vi "clFile_writeToFile.vi"(8 "filename (use dialog)":path, 11 "clFile.lvclass":refnum<class "clFile.lvclass">) -> (3 "no Error":bool)   [LabVIEW 2016, in "vi_lib.lvlib" / "clFile.lvclass"]
uses:
  clFile.lvclass
  clFile.lvclass/clFile.ctl
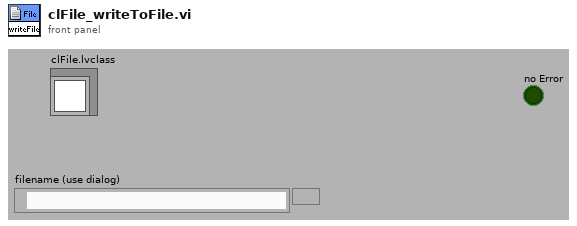
[diagram p1: front panel]
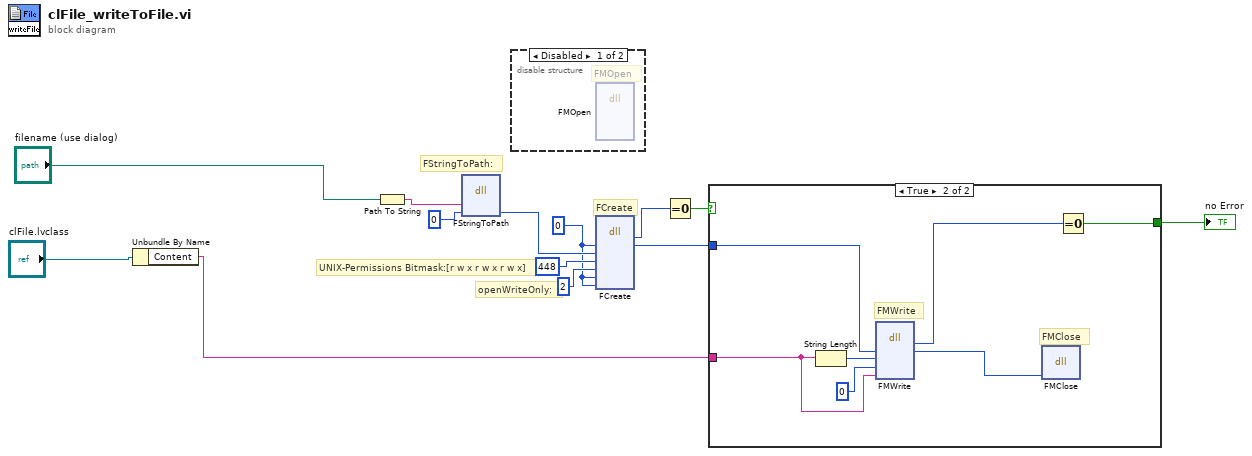
[diagram p0: block diagram]
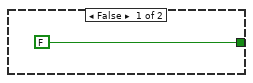
[diagram p2: hidden frame]
diagram:
  w4 = 0 ("denyMode")
  # "FCreate"
  # "FStringToPath:"
  # "UNIX-Permissions Bitmask:[r w x r w x r w x]"
  # "openWriteOnly:"
  n1 = Unbundle By Name("clFile.lvclass") -> ("Content"=w12:string)
  n2 = Path To String(path="filename (use dialog)") -> (string=w8:string)
  n3 = dll-call lib="LabVIEW" fn="FStringToPath"("path"=w8, "pid"=u32 0) -> ("pid"=w7:u32)  [unwired: 4 in, 3 out]
  n4 = disable-structure shown="Disabled" {
    frame Disabled {
      # "FMOpen"
      n5 = dll-call lib="LabVIEW" fn="FMOpen"() -> ()  [unwired: 9 in, 5 out]
    }
    frame Enabled {
    }
  }
  n6 = dll-call lib="LabVIEW" fn="FCreate"("fd"=w4, "path"=w7, "permissions"=448, "openMode"=2, "denyMode"=w4, "group"=w4) -> ("return type"=w2:i32, "fd"=w11:i32)  [unwired: 8 in, 2 out]
  n7 = Equal To 0?(x=w2) -> (x = 0?=w3:bool)
  n8 = case shown="True" w3 {
    tunnel: w12 -> [_ w19]
    tunnel: w11 -> [_ w18]
    tunnel: [FALSE ("OK") w16] -> w1
    frame False {
    }
    frame True {
      # "FMClose"
      # "FMWrite"
      n9 = String Length(string=w19) -> (length=w21:i32)
      n10 = dll-call lib="LabVIEW" fn="FMWrite"("fd"=w18, "inCount"=w21, "outCountp"=0, "buffer"=w19) -> ("return type"=w15:i32, "fd"=w17:i32)  [unwired: 5 in, 3 out]
      n11 = dll-call lib="LabVIEW" fn="FMClose"("fd"=w17) -> ()  [unwired: 4 in, 3 out]
      n12 = Equal To 0?(x=w15) -> (x = 0?=w16:bool)
    }
  }
  "no Error" <- w1
